vi "Test Write Results to DB.vi"   [LabVIEW 2013]
uses:
  Controls/ALTS write DB Result cases.ctl
  Controls/ALTS Write DB Write Result Driver Cases.ctl
  Controls/ALTS LV2GBL Options v1.ctl
types:
  T1 = typedef "ALTS LV2GBL Options v1.ctl" = enum16{"Read all", "Write all"}
  T2 = typedef "ALTS write DB Result cases.ctl" = enum16{"Enter All Data", "Enter WO & SN"}
  T3 = typedef "ALTS Write DB Write Result Driver Cases.ctl" = enum16{"Init", "Write Result", "Close"}
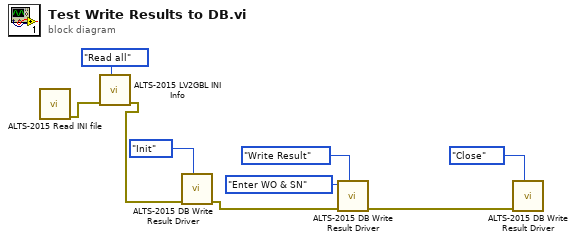
[diagram p0: block diagram]
diagram:
  n1 = call "ALTS-2015 Read INI file.vi"() -> ("error out"=w1:errorcluster)  [unwired: 11 in]
  n2 = call "ALTS-2015 LV2GBL INI Info.vi"("Options"=ALTS_LV2GBL_Options_v1."Read all", "error in"=w1) -> ("error out"=w2:errorcluster)  [unwired: 8 in, 1 out]
  n3 = call "ALTS-2015 DB Write Result Driver.vi"("Operation"=ALTS_Write_DB_Write_Result_Driver_Cases."Init", "Error In"=w2) -> ("error out"=w5:errorcluster)  [unwired: 9 in]
  n4 = call "ALTS-2015 DB Write Result Driver.vi"("Operation"=ALTS_Write_DB_Write_Result_Driver_Cases."Write Result", "Error In"=w5, "DB Write Result Options"=ALTS_write_DB_Result_cases."Enter WO & SN") -> ("error out"=w4:errorcluster)  [unwired: 8 in]
  n5 = call "ALTS-2015 DB Write Result Driver.vi"("Operation"=ALTS_Write_DB_Write_Result_Driver_Cases."Close", "Error In"=w4) -> ()  [unwired: 9 in, 1 out]
